vi "const sourcename.vi"() -> (3 "label":string)   [LabVIEW 2013, in "failure.lvlib"]
uses:
  failure.lvlib
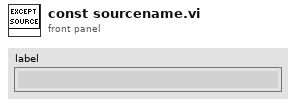
[diagram p1: front panel]
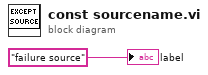
[diagram p0: block diagram]
diagram:
  "label" <- "failure source"
